vi "Parallel Mode Channels Read Single.vi"(8 "error in":errorcluster, 9 "Channel Index":i32=1, 11 "Parallel Mode Channels In":refnum<class "Parallel Mode Channels.lvclass">) -> (0 "error out":errorcluster, 1 "Changed or First Call?":bool, 2 "Parallel Mode Channels ACT":bool, 3 "Parallel Mode Channels Out":refnum<class "Parallel Mode Channels.lvclass">)   [LabVIEW 2023, in "Parallel Mode Channels.lvclass"]
uses:
  Parallel Mode Channels.lvclass
  <vilib>/ADAS Replay HIL/Channels/Tag Wrapper/Tag Wrapper.lvlib
  <vilib>/ADAS Replay HIL/Channels/Tag Wrapper/Polymorphic/Read Channel (Boolean).vi
  693f1d0a-2eeb-4623-aa2b-419758328f6e.vi
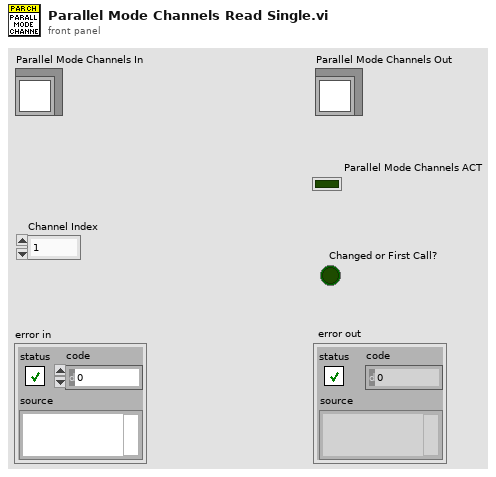
[diagram p1: front panel]
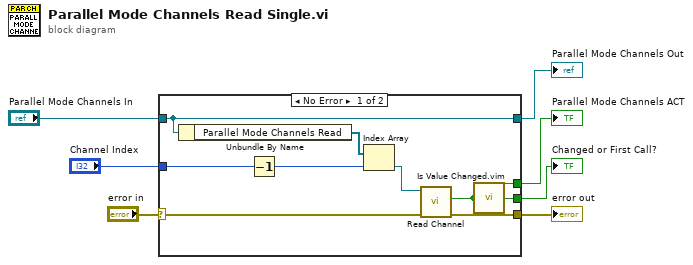
[diagram p0: block diagram]
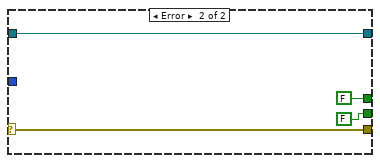
[diagram p2: hidden frame]
diagram:
  n1 = case shown="No Error" "error in" {
    selector: "error in" -> [w14 w20]
    tunnel: [w13 w20] -> w6
    tunnel: [w16 w19] -> w2
    tunnel: "Parallel Mode Channels In" -> [w16 w19]
    tunnel: [w12 FALSE ("Value out")] -> w3
    tunnel: [w11 FALSE ("changed or first call?")] -> w5
    tunnel: "Channel Index" -> [w10 _]
    frame No Error {
      n2 = Unbundle By Name(w16) -> ("Parallel Mode Channels Read"=w15:refnum<k21>[])
      n3 = Decrement(x=w10) -> (x-1=w9:i32)
      n4 = Index Array(array=w15, index=w9) -> (element=w8:refnum<k21>)
      n5 = call-poly <vilib>:"Read Channel.vi"("error in"=w14, "ADAS HIL Channel in"=w8) -> ("error out"=w13:errorcluster, "Value out"=w12:bool)  [unwired: 6 in, 2 out]
      n6 = call "Is Value Changed.vim"("value"=w12) -> ("changed or first call?"=w11:bool)
    }
    frame Error {
    }
  }
  "error out" <- w6
  "Changed or First Call?" <- w5
  "Parallel Mode Channels ACT" <- w3
  "Parallel Mode Channels Out" <- w2
